vi "Set Salida.vi"(8 "error in (no error)":errorcluster, 10 "Array":bool[](array[boolean]), 11 "VISA resource name":refnum<visa-resource-name>) -> (0 "error out":errorcluster, 3 "VISA resource name out":refnum<visa-resource-name>)   [LabVIEW 2014, in "CAP-USB.lvlib"]
doc: "REALIZA LA CONVERSION\nPARA ESCRIBIR LA DIRECCION DE MEMORIA\nY ACTUALIZAR LAS SALIDAS"
uses:
  CAP-USB.lvlib
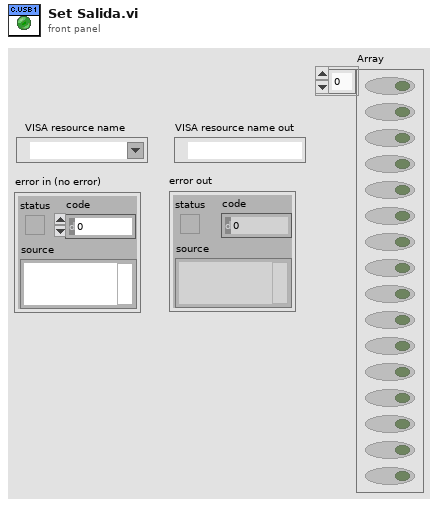
[diagram p1: front panel]
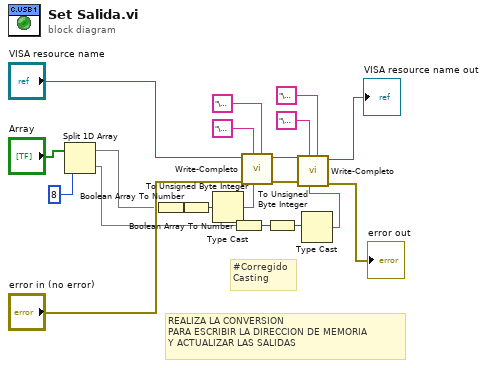
[diagram p0: block diagram]
diagram:
  # "#Corregido\nCasting"
  # "REALIZA LA CONVERSION\nPARA ESCRIBIR LA DIRECCION DE MEMORIA\nY ACTUALIZAR LAS SALIDAS"
  n1 = Split 1D Array(array="Array", index=8) -> (first subarray=w10:bool[], second subarray=w9:bool[])
  n2 = Boolean Array To Number(Boolean array=w10) -> (number=w4:u32)
  n3 = To Unsigned Byte Integer(number=w4) -> (unsigned 8bit integer=w3:u8)
  n4 = Type Cast(x=w3) -> (*(type *) &x=w5:string)  [unwired: 1 in]
  n5 = Boolean Array To Number(Boolean array=w9) -> (number=w2:u32)
  n6 = call "Write-Completo.vi"("Low Byte"="\u0001" ("Hi Byte"), "Dato 8 bits"=w5, "Hi Byte"="\u0003", "error in (no error)"="error in (no error)", "VISA resource name"="VISA resource name") -> ("error out"=w16:errorcluster, "VISA resource name out"=w15:refnum<visa-resource-name>)  [unwired: 5 in]
  n7 = To Unsigned Byte Integer(number=w2) -> (unsigned 8bit integer=w1:u8)
  n8 = Type Cast(x=w1) -> (*(type *) &x=w6:string)  [unwired: 1 in]
  n9 = call "Write-Completo.vi"("Low Byte"="\u0005" ("Hi Byte"), "Dato 8 bits"=w6, "Hi Byte"="\u0003", "error in (no error)"=w16, "VISA resource name"=w15) -> ("error out"=→"error out":errorcluster, "VISA resource name out"=→"VISA resource name out":refnum<visa-resource-name>)  [unwired: 5 in]
